vi "Finalización_VBombas.vi"(0 "Refnum in":refnum<k21>, 5 "error in (no error)":errorcluster) -> (19 "error out":errorcluster)   [LabVIEW 2013]
uses:
  <vilib>/DAQmx/write.llb/DAQmx Write (Analog DBL 1Chan 1Samp).vi
  <vilib>/DAQmx/miscellaneous.llb/DAQmx Fill In Error Info.vi
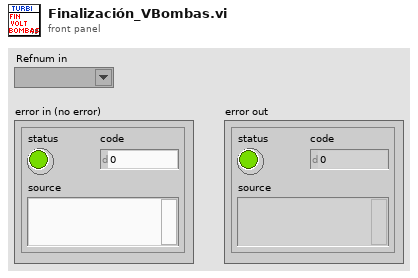
[diagram p1: front panel]
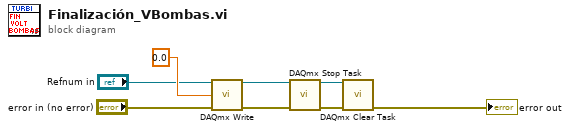
[diagram p0: block diagram]
diagram:
  n1 = call-poly <vilib>:"DAQmx Write.vi"("task/channels in"="Refnum in", "data"=0.0, "error in"="error in (no error)") -> ("task out"=w5:refnum<k21>, "error out"=w4:errorcluster)  [unwired: 10 in, 1 out]
  n2 = call <vilib>:"DAQmx Stop Task.vi"("task/channels in"=w5, "error in"=w4) -> ("task out"=w3:refnum<k21>, "error out"=w2:errorcluster)  [unwired: 12 in]
  n3 = call <vilib>:"DAQmx Clear Task.vi"("task in"=w3, "error in"=w2) -> ("error out"=→"error out":errorcluster)  [unwired: 13 in]
